vi "Set Seqence.vi"(8 "Error In":errorcluster, 10 "Iteration":i32, 11 "Power Seq":T1=[{"Duration"=10, "Head Load(W)"=100, "Name"="Step1"}, {"Duration"=60, "Head Load(W)"=150, "Name"="Step2"}, {"Duration"=120, "Head Load(W)"=50, "Name"="Step3"}]) -> (0 "Error Out":errorcluster, 3 "Waveform Graph":u32[](graph))   [LabVIEW 2019, in "GUI.lvlib"]
uses:
  GUI.lvlib
  Controls/Profile Sequence.ctl
panel:
  # "Step"
  # "Duration"
  # "Heat Load(W)"
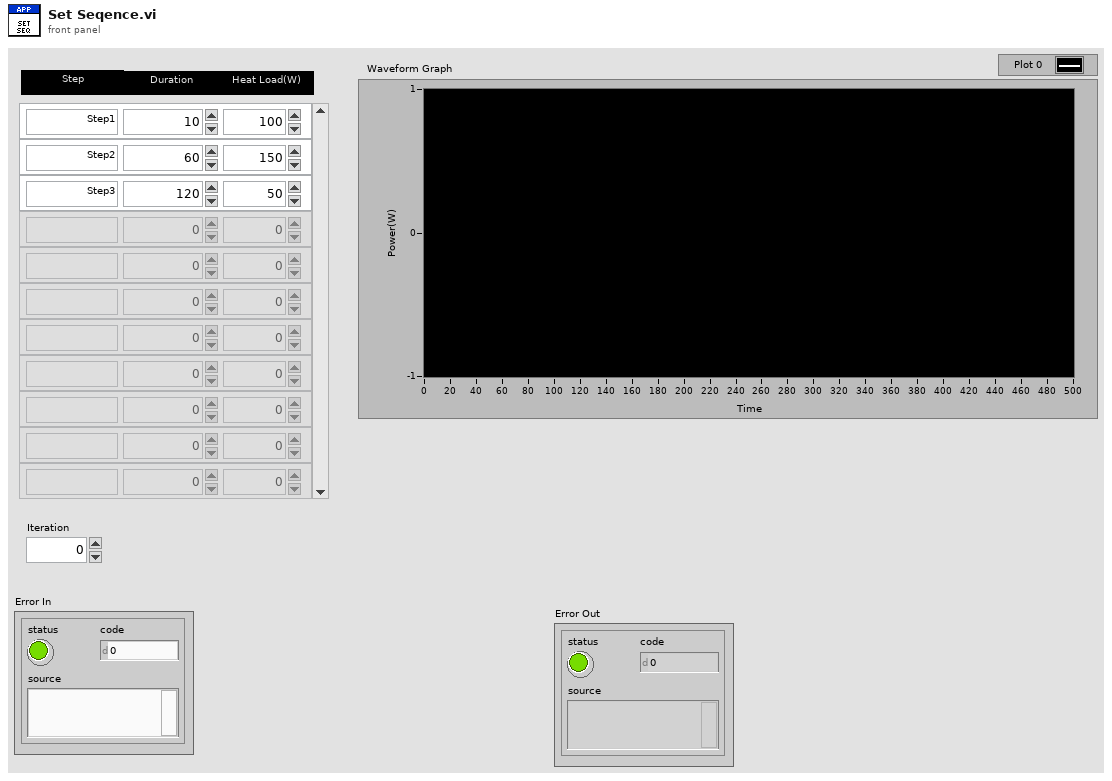
[diagram p1: front panel]
types:
  T1 = typedef "GUI.lvlib/Profile Sequence.ctl" = cluster{"Duration":i32, "Head Load(W)":u32, "Name":string}[]
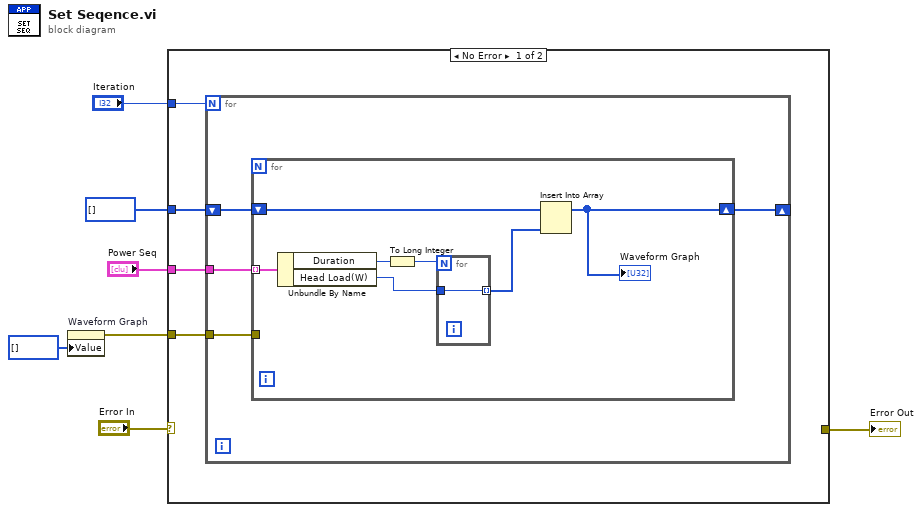
[diagram p0: block diagram]
diagram:
  n1 = property on="Waveform Graph" class="WFGraph (strict)"("Value"=u32[] [] ("Waveform Graph")) -> (error out=w6:errorcluster)  [unwired: 2 in, 1 out]
  n2 = case shown="No Error" "Error In" {
    selector: "Error In" -> [_ w24]
    tunnel: "Power Seq" -> [w11 _]
    tunnel: w6 -> [w10 _]
    tunnel: u32[] [] -> [w9 _]
    tunnel: [_ w24] -> w4
    tunnel: "Iteration" -> [w8 _]
    frame No Error {
      n3 = for {
        N: w8 -> [_]
        tunnel: w11 -> [w15]
        tunnel: w10 -> [w14]
        shift-right: [w12] -> _
        shift-left: w9 -> [w13]
        n4 = for {
          tunnel: w15 -> [w22] mode=indexing
          tunnel: w14 -> [_]
          shift-right: [w16] -> w12
          shift-left: w13 -> [w21]
          n5 = Unbundle By Name(w22) -> ("Duration"=w20:i32, "Head Load(W)"=w19:u32)
          n6 = To Long Integer(number=w20) -> (32bit integer=w18:i32)
          n7 = for {
            N: w18 -> [_]
            tunnel: w19 -> [w23]
            tunnel: [w23] -> w17 mode=indexing
          }
          n8 = Insert Into Array(array=w21, new element=w17) -> (w16:u32[])  [unwired: 1 in]
          "Waveform Graph" <- w16
        }
      }
    }
    frame Error {
    }
  }
  "Error Out" <- w4
